vi "Parse callibration info.vi"(0 "Refnum in":T1, 1 "Statistics in":T2, 2 "server url in":string, 3 "error in (no error)":errorcluster) -> (6 "Refnum out":T1, 7 "Statistics out":T2, 9 "error out":errorcluster)   [LabVIEW 2020]
uses:
  <vilib>/httpClient/ClientHandle.ctl
  <vilib>/httpClient/LabVIEWHTTPClient.lvlib
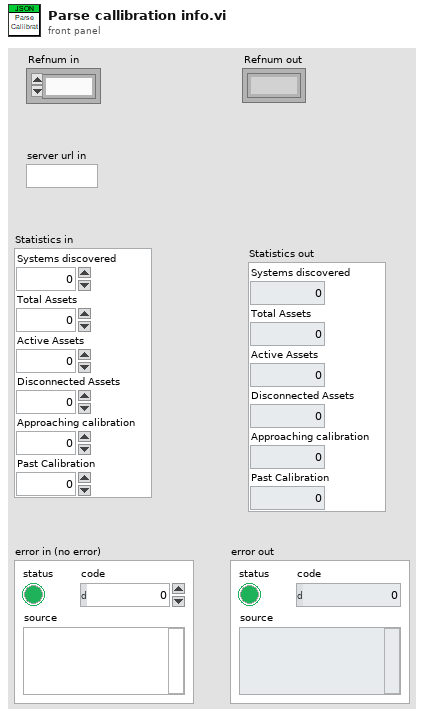
[diagram p1: front panel]
types:
  T1 = typedef "LabVIEWHTTPClient.lvlib/ClientHandle.ctl" = refnum<k1>
  T2 = cluster{"Systems discovered":i32, "Total Assets":i32, "Active Assets":i32, "Disconnected Assets":i32, "Approaching calibration ":i32, "Past Calibration":i32}
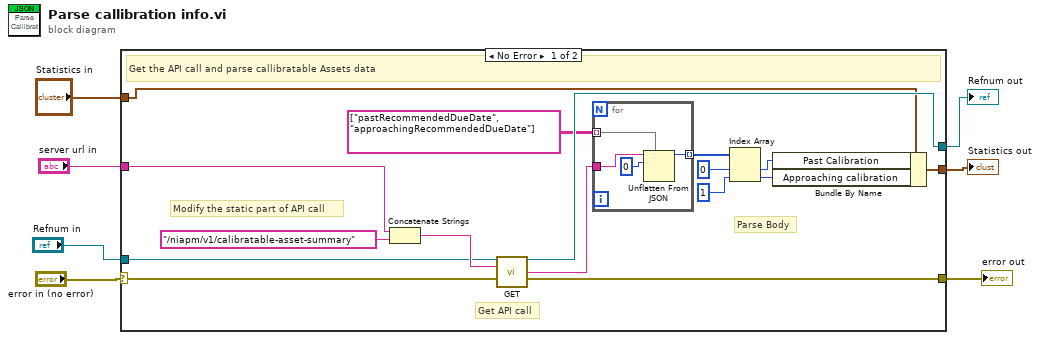
[diagram p0: block diagram]
diagram:
  n1 = case shown="No Error" "error in (no error)" {
    selector: "error in (no error)" -> [w9 w29]
    tunnel: "server url in" -> [w23 _]
    tunnel: [w22 w29] -> w6
    tunnel: [w21 w30] -> w5
    tunnel: [w18 w28] -> w4
    tunnel: "Statistics in" -> [w17 w28]
    tunnel: "Refnum in" -> [w10 w30]
    frame No Error {
      # "Parse Body"
      # "Get API call"
      # "Modify the static part of API call"
      # "Get the API call and parse callibratable Assets data"
      n2 = Concatenate Strings(w23, "/niapm/v1/calibratable-asset-summary" ("Amount of calibratable assets")) -> (w12:string)
      n3 = call <vilib>:"GET.vi"("client handle"=w10, "url"=w12, "error in (no error)"=w9) -> ("client handle out"=w21:T1, "body"=w8:string, "error out"=w22:errorcluster)  [unwired: 9 in, 1 out]
      n4 = for {
        tunnel: [w26] -> w13 mode=indexing
        tunnel: string[][] [["pastRecommendedDueDate"], ["approachingRecommendedDueDate"]] -> [w25] mode=indexing
        tunnel: w8 -> [w24]
        n5 = Unflatten From JSON(path=w25, JSON string=w24, type and defaults=0) -> (value=w26:i32)  [unwired: 4 in, 1 out]
      }
      n6 = Index Array(array=w13, index #1=0 ("index"), index #2=1 ("index")) -> (element #1=w19:i32, element #2=w20:i32)
      n7 = Bundle By Name(cluster=w17, "Past Calibration"=w19, "Approaching calibration"=w20) -> (w18:T2)
    }
    frame Error {
    }
  }
  "error out" <- w6
  "Refnum out" <- w5
  "Statistics out" <- w4
